vi "Close_Task.vi"(8 "error in (no error)":errorcluster caption="entrée d'erreur (pas d'erreur)", 11 "Class Log_File (Default) en entrée":refnum<class "Class Log_File (Default).lvclass">) -> (0 "error out":errorcluster caption="sortie d'erreur", 3 "Class Log_File (Default) en sortie":refnum<class "Class Log_File (Default).lvclass">)   [LabVIEW 2020, in "Library Instrument & Equipement.lvlib" / "Library Log_File.lvlib" / "Class Log_File (Default).lvclass"]
uses:
  Class Log_File (Default).lvclass
  Class Log_File (Default).lvclass/Class Log_File (Default).ctl
  Read CSV File/CSV_File (Default)/Class CSV_File.lvclass
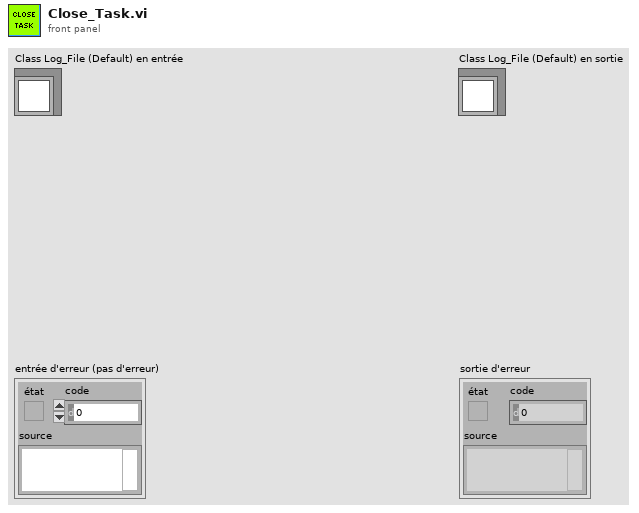
[diagram p1: front panel]
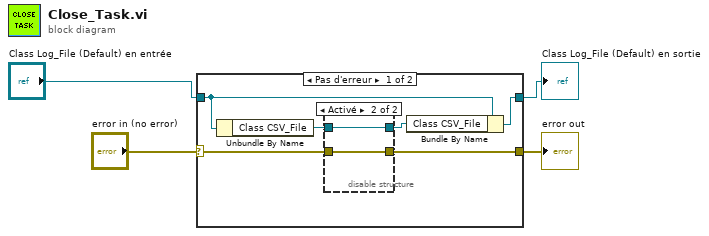
[diagram p0: block diagram]
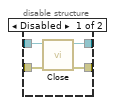
[diagram p2: hidden frame]
diagram:
  n1 = case shown="Pas d'erreur" "error in (no error)" {
    selector: "error in (no error)" -> [w10 w18]
    tunnel: [w9 w18] -> w3
    tunnel: [w6 w17] -> w1
    tunnel: "Class Log_File (Default) en entrée" -> [w5 w17]
    frame No Error {
      n2 = Unbundle By Name(w5) -> ("Class CSV_File"=w8:refnum<class "Class CSV_File.lvclass">)
      n3 = disable-structure shown="Activé" {
        disable-tunnel: w10 -> [w14 w15]
        disable-tunnel: [w13 w15] -> w9
        disable-tunnel: w8 -> [w12 w16]
        disable-tunnel: [w11 w16] -> w7
        frame Disabled {
          n4 = call-dynamic "Close.vi"("error in (no error)"=w14, "Class CSV_File (Default) en entrée"=w12) -> ("error out"=w13:errorcluster, "Class CSV_File (Default) en sortie"=w11:refnum<class "Class CSV_File.lvclass">)  [unwired: 8 in]
        }
        frame Enabled {
        }
      }
      n5 = Bundle By Name(cluster=w5, "Class CSV_File"=w7) -> (w6:refnum<class "Class Log_File (Default).lvclass">)
    }
    frame Error {
    }
  }
  "error out" <- w3
  "Class Log_File (Default) en sortie" <- w1
